vi "sub_isDrawGame.vi"(11 "array":string[](array[string])) -> (3 "is draw":bool)   [LabVIEW 2018]
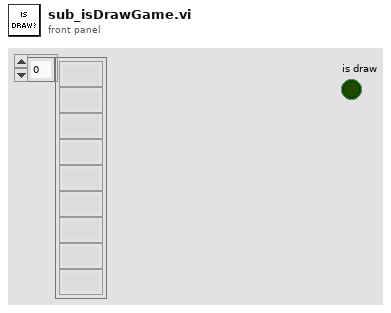
[diagram p1: front panel]
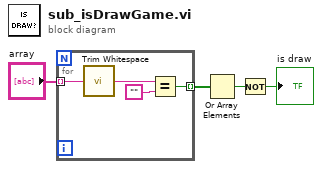
[diagram p0: block diagram]
diagram:
  n1 = for {
    tunnel: "array" -> [w8] mode=indexing
    tunnel: [w5] -> w3 mode=indexing
    n2 = call <vilib>:"Trim Whitespace.vi"("string"=w8) -> ("trimmed string"=w7:string)  [unwired: 1 in]
    n3 = Equal?(x=w7, y="") -> (x = y?=w5:bool)
  }
  n4 = Or Array Elements(Boolean array=w3) -> (logical OR=w2:bool)
  n5 = Not(x=w2) -> (.not. x?=→"is draw":bool)
